vi "LabelImage.vi"(7 "Mode?":enum16{"Overlay", "Extend"}(ring), 8 "error in (no error)":errorcluster, 9 "Label":string, 10 "Original image in":T1, 11 "Labeled image in":T1) -> (0 "error out":errorcluster, 2 "Original image out":T1, 3 "Labeled image out":T1)   [LabVIEW 2012]
uses:
  <vilib>/vision/Image Controls.llb/IMAQ Image.ctl
  <vilib>/vision/NI_Vision_Development_Module.lvlib
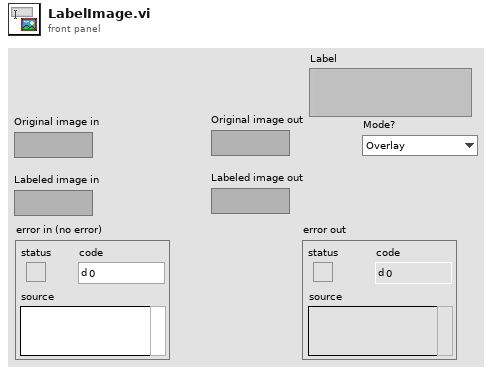
[diagram p1: front panel]
types:
  T1 = typedef "IMAQ Image.ctl" = refnum<image>
  T2 = enum16{"User-specified Font", "Application Font", "System Font", "Dialog Font"}
  T3 = cluster{"Font Name":string, "Size":i16, "Strikeout?":bool, "Italic?":bool, "Underline?":bool, "Outline?":bool, "Shadow?":bool, "Bold?":bool, "Rotation Angle":dbl}
  T4 = cluster{"Desired Font (Application)":enum16{"User-specified Font", "Application Font", "System Font", "Dialog Font"}, "[User-specified Font]":cluster{"Font Name":string, "Size":i16, "Strikeout?":bool, "Italic?":bool, "Underline?":bool, "Outline?":bool, "Shadow?":bool, "Bold?":bool, "Rotation Angle":dbl}, "Horizontal Alignment":i16, "Vertical Alignment":i16}
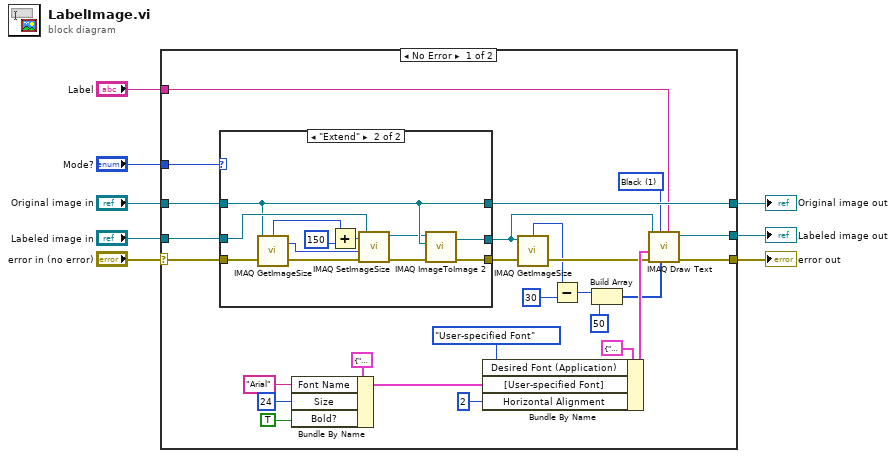
[diagram p0: block diagram]
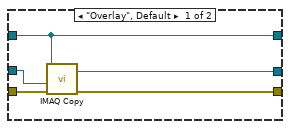
[diagram p2: hidden frame]
diagram:
  n1 = case shown="No Error" "error in (no error)" {
    selector: "error in (no error)" -> [w31 w52]
    tunnel: "Mode?" -> [w34 _]
    tunnel: "Original image in" -> [w33 w54]
    tunnel: "Labeled image in" -> [w32 w53]
    tunnel: [w30 w54] -> w4
    tunnel: [w28 w52] -> w3
    tunnel: [w27 w53] -> w2
    tunnel: "Label" -> [w19 _]
    frame No Error {
      w11 = 1 items=["White", "Black", "Inverted", "Black on White", "White on Black"] ("Color")
      n2 = case shown="\"Extend\"" w34 {
        tunnel: w33 -> [w35 w41]
        tunnel: w32 -> [w38 w44]
        tunnel: w31 -> [w39 w51]
        tunnel: [w37 w42] -> w17
        tunnel: [w36 w43] -> w29
        tunnel: [w35 w41] -> w30
        frame "Overlay", Default {
          n3 = call "IMAQ Copy"("error in (no error)"=w39, "Image Dst"=w38, "Image Src"=w35) -> ("error out"=w36:errorcluster, "Image Dst Out"=w37:T1)  [unwired: 3 in]
        }
        frame "Extend" {
          n4 = call "IMAQ GetImageSize"("Image"=w41, "error in (no error)"=w51) -> ("Y Resolution"=w49:i32, "X Resolution"=w47:i32, "error out"=w50:errorcluster)  [unwired: 2 in]
          n5 = Add(x=w47, y=150) -> (x+y=w48:i32)
          n6 = call "IMAQ SetImageSize"("error in (no error)"=w50, "Y Resolution"=w49, "X Resolution"=w48, "Image"=w44) -> ("error out"=w45:errorcluster, "Image Out"=w40:T1)  [unwired: 1 in]
          n7 = call "IMAQ ImageToImage 2"("error in (no error)"=w45, "Image Src (Small)"=w41, "Image Src (Large)"=w40) -> ("error out"=w43:errorcluster, "Image Dst Out"=w42:T1)  [unwired: 7 in]
        }
      }
      n8 = Bundle By Name(cluster=T3 {"Font Name"="", "Size"=0, "Strikeout?"=FALSE, "Italic?"=FALSE, "Underline?"=FALSE, "Outline?"=FALSE, "Shadow?"=FALSE, "Bold?"=FALSE, "Rotation Angle"=0.0} ("[User-specified Font]"), "Font Name"="Arial", "Size"=i16 24, "Bold?"=TRUE) -> (w23:T3)
      n9 = Bundle By Name(cluster=T4 {"Desired Font (Application)"=enum."Application Font", "[User-specified Font]"={"Font Name"="", "Size"=12, "Strikeout?"=FALSE, "Italic?"=FALSE, "Underline?"=FALSE, "Outline?"=FALSE, "Shadow?"=FALSE, "Bold?"=FALSE, "Rotation Angle"=0.0}, "Horizontal Alignment"=0, "Vertical Alignment"=0} ("Font, Size & Style"), "Desired Font (Application)"=T2."User-specified Font", "[User-specified Font]"=w23, "Horizontal Alignment"=i16 2) -> (w25:T4)
      n10 = call "IMAQ GetImageSize"("Image"=w17, "error in (no error)"=w29) -> ("X Resolution"=w16:i32, "error out"=w18:errorcluster)  [unwired: 2 in, 1 out]
      n11 = Subtract(x=w16, y=30) -> (x-y=w14:i32)
      n12 = Build Array(w14, 50 ("element")) -> (w12:i32[])
      n13 = call "IMAQ Draw Text"("String"=w19, "Insertion Point"=w12, "Color"=w11, "error in (no error)"=w18, "Font, Size & Style"=w25, "Image Src"=w17) -> ("error out"=w28:errorcluster, "Image Dst Out"=w27:T1)  [unwired: 2 in, 2 out]
    }
    frame Error {
    }
  }
  "Original image out" <- w4
  "error out" <- w3
  "Labeled image out" <- w2
